vi "HFRR ADV v09.vi"() -> ()   [LabVIEW 2025] (continued)
18.549185433725157, 18.540397690756503, 18.52985239919411, 18.52985239919411, 18.5122769132568, 18.51403446185053, 18.515792010444265, 18.482398587163367, 18.494701427319487, 18.475368392788447, 18.464823101226052, 18.443732518101285, 18.459550455444862, 18.44900516388247, 18.427914580757704, 18.45076271247621, 18.436702323726358, 18.42439948357024, 18.433187226538898, 18.427914580757704, 18.408581546226657, 18.41385419200785, 18.389248511695616, 18.398036254664273, 18.38573341450815, 18.38221831732069, 18.38221831732069, 18.35058244263353, 18.368157928570838, 18.348824894039797, 18.34706734544607, 18.340037151071144, 18.331249408102487, 18.327734310915027, 18.31543147075891, 18.31543147075891, 18.301371082009055, 18.287310693259204, 18.297855984821588, 18.280280498884274, 18.275007853103087, 18.269735207321887, 18.25567481857205, 18.252159721384576, 18.232826686853535, 18.239856881228466, 18.215251200916224, 18.217008749509954, 18.209978555135034, 18.19064552060399, 18.195918166385184, 18.183615326229067, 18.169554937479216, 18.17307003466668, 18.153737000135635, 18.151979451541898, 18.137919062792054, 18.125616222635934, 18.12737377122967, 18.115070931073546, 18.115070931073546, 18.10276809091743, 18.099252993729966, 18.095737896542506, 18.09046525076131, 18.081677507792655, 18.067617119042804, 18.062344473261614, 18.055314278886687, 18.044768987324296, 18.03598124435564, 18.032466147168176, 18.023678404199522, 18.025435952793252, 18.021920855605796, 18.00961801544967, 17.99907272388729, 17.997315175293558, 17.99204252951236, 17.98501233513744, 17.97095194638759, 17.963921752012663, 17.958649106231476, 17.953376460450276, 17.946346266075352, 17.934043425919235, 17.93580097451296, 17.97095194638759, 17.953376460450276, 17.955134009044006, 17.94283116888789, 17.93931607170043, 17.927013231544308, 17.921740585763114, 17.891862259669683, 17.895377356857146, 17.89889245404461, 17.893619808263416, 17.881316968107296, 17.88307451670103, 17.879559419513566, 17.865499030763715, 17.833863156076553, 17.837378253264013, 17.80925747576432, 17.796954635608202, 17.796954635608202, 17.78465179545208, 17.77234895529596, 17.767076309514763, 17.777621601077154, 17.774106503889694, 17.742470629202533, 17.768833858108493, 17.719622497484025, 17.724895143265222, 17.724895143265222, 17.7178649488903, 17.728410240452682, 17.707319657327908, 17.70028946295298, 17.716107400296565, 17.703804560140444, 17.677441331234476, 17.65107810232851, 17.66865358826582, 17.5772610613918, 17.53859499232971, 17.52277705498613, 17.52453460357986, 17.515746860611202, 17.51047421483001, 17.50871666623628, 17.49992892326762, 17.491141180298964, 17.480595888736577, 17.477080791549124, 17.466535499986733, 17.464777951393007, 17.45423265983061, 17.44720246545569, 17.43314207670584, 17.43489962529957, 17.43138452811211, 17.419081687955984, 17.4085363963936, 17.403263750612407, 17.403263750612407, 17.390960910456286, 17.38744581326883, 17.382173167487633, 17.368112778737785, 17.368112778737785, 17.35405238998793, 17.347022195613008, 17.34174954983182, 17.339992001238087, 17.329446709675697, 17.325931612488237, 17.31714386951958, 17.308356126550922, 17.304841029363462, 17.303083480769722, 17.29429573780107, 17.278477800457495, 17.2732051546763, 17.26969005748884, 17.26265986311391, 17.257387217332717, 17.252114571551527, 17.245084377176603, 17.239811731395402, 17.23805418280167, 17.223993794051825, 17.223993794051825, 17.22047869686436, 17.213448502489445, 17.209933405301975, 17.20290321092705, 17.192357919364667, 17.188842822177204, 17.178297530614817, 17.17478243342735, 17.15720694749004, 17.146661655927648, 17.14490410733392, 17.136116364365265, 17.12908616999034, 17.122055975615414, 17.113268232646764, 17.178297530614817, 17.162479593271232, 17.115025781240494, 17.08338990655333, 17.081632357959595, 17.081632357959595, 17.067571969209745, 17.067571969209745, 17.06054177483482, 17.05702667764736, 17.051754031866164, 17.042966288897507, 17.035936094522594, 17.02363325436647, 17.01484551139781, 17.00957286561662, 16.995512476866768, 16.991997379679308, 16.990239831085574, 16.98496718530438, 16.979694539523184, 16.977936990929454, 16.96387660217961, 16.95508885921095, 16.951573762023486, 16.94278601905482, 16.933998276086164, 16.933998276086164, 16.92169543593005, 16.91642279014886, 16.9129076929614, 16.91642279014886, 16.904119949992744, 16.897089755617817, 16.895332207024087, 16.88654446405543, 16.87775672108677, 16.883029366867966, 16.867211429524385, 16.858423686555728, 16.85490858936826, 16.846120846399604, 16.832060457649764, 16.83030290905603, 16.823272714681107, 16.81624252030618, 16.810969874524982, 16.802182131556325, 16.8004245829626, 16.789879291400208, 16.789879291400208, 16.781091548431554, 16.768788708275437, 16.770546256869167, 16.767031159681704, 16.756485868119317, 16.754728319525583, 16.745940576556933, 16.738910382182006, 16.733637736400812, 16.724849993432162, 16.716062250463505, 16.702001861713647, 16.69672921593246, 16.698486764526187, 16.684426375776336, 16.682668827182606, 16.677396181401413, 16.666850889839022, 16.661578244057836, 16.659820695464106, 16.64927540390171, 16.640487660933058, 16.633457466558134, 16.628184820776944, 16.622912174995744, 16.622912174995744, 16.615881980620824, 16.60533668905843, 16.600064043277243, 16.59830649468351, 16.5807310087462, 16.577215911558728, 16.573700814371275]
  in  "ENTER THE NEW PASSWORD":string caption="Enter The New Password"
  in  "ENTER CURRENT PASSWORD":string caption="Enter Current Password"
  in  "Camera Port :":string(combo)="cam0"
  in  "Humidity :":refnum<visa-resource-name>="COM8"
  in  "LvdtOff":dbl=2.875 caption="LVDT Position Offset :" min=2.1 max=2.9 format="%.4f"
  out "Port 2 Error":errorcluster={"status"=TRUE, "code"=-1073807343, "source"="Property Node (arg 1) in VISA Configure Serial Port (Instr).vi->Winducom 2010--std ed hfrr-wo1768-V18.vi"}
  out "Port 1 Error":errorcluster={"status"=TRUE, "code"=-1073807343, "source"="Property Node (arg 1) in VISA Configure Serial Port (Instr).vi->Winducom 2010--std ed hfrr-wo1768-V18.vi"}
  in  "Stroke PID Gains":T8={"Proportional Gain (Kc)"=200.0, "Integral Time (Ti, min)"=0.02, "Derivative Time (Td, min)"=0.0}
  in  "CH-HUMIDITY DRY":u16=3 caption="Ch-Humidity Wet:" max=7 step=1
  in  "CH-HUMIDITY WET":u16=4 caption="Ch-Humidity Dry:" max=7 step=1
  in  "CH-HEATER":u16=2 caption="Ch-Heater:" max=7 step=1
  in  "CH-POWER -":u16=1 caption="Ch-Power -:" max=7 step=1
  in  "CH-POWER +":u16 caption="Ch-Power +:" max=7 step=1
  out "String 4":string
  in  "Prog Due":bool
  in  "Prog Uno":bool
  in  "Com Port 2":refnum<visa-resource-name>="COM7" caption="Port 2 :"
  in  "Com Port 1":refnum<visa-resource-name>="COM5" caption="Port 1 :"
  in  "Additional Parameter":T9(tab)
  out "CAMERA ROI MIN TEMP":bool
  in  "CAMERA ROI MAX TEMP":bool
  out "LIVE FEED MIN TEMP":bool
  in  "LIVE FEED MAX TEMP":bool
  in  "Temperature Off Command":bool
  in  "Temperature On Command":bool
  in  "Humidity Off Command":bool
  in  "Humidity On Command":bool
  out "Elapsed time":dbl caption="Elapsed Time" min=0.0 max=6000.0 step=0.01 format="%.2f"
  in  "Remaining Time":dbl min=0.0 max=180000.0 step=0.0001 format="%<%H:%M:%S>t"
  out "Auto Start Temp":bool
  out "Auto stop temp":bool
  in  "TestCompFlg":bool
  out "StartFlg":bool
  in  "Start Time":bool
  in  "sign in temp":bool
  in  "manual temp log":bool
  in  "Reach point temp":bool
  in  "Manual Humididty Reached":bool
  out "Humidity temp":dbl
  in  "Test ID":string
  in  "Reach point Humidity":bool
  in  "error in (no error) 2":errorcluster
  out "Instrument Status":bool=TRUE caption="Load COM Status"
  out "Heave Pulses/mm":dbl=1600.0
  out "Surge Pulses/mm":dbl=1600.0
  out "Sway Pulses/mm":dbl=320.0
  in  "Surge Pitch":dbl=3.0
  in  "Sway Pitch":dbl=2.0
  in  "Heave Pitch":dbl=4.0
  in  "Surge PPR":dbl=6400.0
  in  "Sway PPR":dbl=6400.0
  in  "Heave PPR":dbl=6400.0
  in  "Heater Trip Temp":bool
  out "String 41":string=":-@(Paltro : HIGH FREQUENCY RECIPROCATORY TEST RIG    DEFINITON FILE )      "
  out "Service Password enable":bool
  out "TEST FILE NAM,E SAVED":bool
  out "error out 6":errorcluster
  out "error out 7":errorcluster
  out "error out 8":errorcluster
  out "Camera List":string
  out "Image path  2":path caption="selected path"
  out "100x gain":dbl
  out "Pixel Value":dbl
  in  "Enum - Selector":T10
  out "Image path":path
  out "Error":errorcluster={"status"=TRUE, "code"=-1073807343, "source"="Property Node (arg 1) in VISA Configure Serial Port (Instr).vi->Winducom 2010--std ed hfrr-wo1768-V18.vi"}
  out "Bytes at Humidity Port":dbl
  in  "Com Port 4":refnum<visa-resource-name>="COM7" caption="COM Port Humidity :"
  out "Read Humidity":string
  in  "String 11":string
  in  "WriteHumidity":string[](array[string])
  out "LastCom":string
  in  "Write S":bool
  out "STALL :":string
  out "CURRENT :":string
  out "DEHUM :":string
  out "FAN_OUT :":string
  out "FAN_IN :":string
  out "PUMP :":string
  out "AMB_T :":string
  out "AMB_RH :":string
  out "T :":string
  out "RH :":string
  out "SET :":string
  out "STATE :":string
  out "RH Numeric:":dbl
  out "COM Status":bool=TRUE caption="Load COM Status"
  in  "Tab Control 6":enum32{"Data", "Sensor"}(tab)=enum."Sensor"
  out "Respose From Server":string
  out "standard output":string
  out "SinglePoint":string
  in  "JSON Check String":string="\"Stored\": true"
  in  "JSONH Check String":string="\"Stored\": true"
  out "standard output 2":string
  in  "Sensor Information":string[][](array[string])=[["Sensor Name", "Sensor Model Number", "Sensor Run time Hours", "Sensor State"], ["Normal Load Sensor", "MPF-AC20-X3U791", "", ""], ["Frictional Force Sensor", "MPF-AC20-X3U792", "", ""], ["Temperature Sensor", "MPF-AC20-X3U793", "", ""], ["Speed Sensor", "MPF-AC20-X3U794", "", ""], ["LVDT Sensor", "MPF-AC20-X3U795", "", ""], ["Vibration Sensor ", "MPF-AC20-X3U796", "", ""]]
  out "Respose From Server 2":string
  in  "Total No. of Tests":dbl
  in  "Upld AR":bool
  in  "Sensor File Name":string="JSON_Health.JSON"
  in  "Run test 3":bool
  in  "Sen.Upload Rate (s)":dbl=5.0 min=0.5 max=5.0 step=0.5 format="%.1g"
  in  "Upld AR 2":bool
  in  "Path":path=path "C:/LAB-IQ-NXT"
  in  "Data File Name":string="JSON_Single_Point.JSON"
  in  "Model No":string="MD987654325"
  in  "Serial No":string="HFRR2391"
  in  "Secret Key":string="22gKHnAGFaJhuNtaR9srYhcD6RQR8M7Zp2xk4ssPTuwGqWUBv7WxW7cXAFkFFbns"
  in  "Upload Rate (s)":dbl=1.0 min=0.5 max=5.0 step=0.5 format="%.1g"
  in  "ADC Res":u16(ring) items=["16 bit", "24 bit"]
  out "Test Standard":string
  out "error out 5":errorcluster
  out "after substring":string
  out "before substring 2":string
  in  "Temperature after test 3":dbl caption="Temp After Test" format="%#_5g"
  in  "Humidity after test 3":dbl caption="Humidity After Test" format="%#_5g"
  in  "Tab Control 4":T11(tab)=enum."Temperature Tuning"
  in  "ECR_Gain":dbl=24000.0
  out "Ch3 2":dbl[](graph)
  out "Air temp":dbl[](graph)
  out "ECR":dbl[](graph)
  out "Rtemp":dbl[](graph)
  in  "Do 0":bool
  out "DI 0":bool=TRUE
  out "DI 1":bool=TRUE
  out "DI 2":bool=TRUE
  out "DI 3":bool=TRUE
  out "DI 4":bool=TRUE
  out "DI 5":bool=TRUE
  out "DI 6":bool=TRUE
  out "DI 7":bool=TRUE
  in  "Do 7":bool
  in  "Do 6":bool
  in  "Do 5":bool
  in  "Do 4":bool
  in  "Do 3":bool
  in  "Do 2":bool
  in  "Do 1":bool
  in  "output range":cluster{"output high":dbl, "output low":dbl}={"output high"=110.0, "output low"=0.0}
  in  "Offset Air Temp":dbl
  in  "Temp PID gains":T12={"proportional gain (Kc)"=10.0, "integral time (Ti, min)"=1.66, "derivative time (Td, min)"=0.0}
  out "gTEMP 3":cluster{dbl, "output":dbl, "Set Temp":dbl}(graph)={6.858462627117447, "output"=42.16277107130474, "Set Temp"=53.14153737288255}
  out "Pk-Pk":dbl=0.5
  in  "Offset":dbl=0.5
  in  "Gain":dbl=1.4
  out "gLVDTraw":dbl[](graph)
  out "Disp":dbl=-1.7485910993892546e-16 caption="Stroke" format="%.2f"
  out "Freq":dbl=50.0 caption="Frequency" min=10.0 max=250.0 step=0.1 format="%.2f"
  out "PID Out":u8(slide) scale=0.0..4095.0
  out "Freq":dbl min=0.0 max=12.0 step=0.01 format="%.3f"
  out "Array":string[](array[string])
  out "UnoRead":string
  out "Sps 2":dbl=890.0 format="%_0f"
  out "Disp (mm)":dbl=1.0 min=0.0 max=12.0 step=0.01 format="%.3f"
  in  "PID Rst":bool=TRUE
  in  "DC correction":bool=TRUE
  out "Mean(RAW) Stroke":dbl(graph)
  out "Waveform Graph 2":waveform(dbl)[](graph)
  out "Stroke PID OUT":dbl(slide)=-13.483146067415703 scale=-600.0..600.0
  out "Slide 8":cluster{dbl, dbl, dbl}(slide)={-13.483146067415703, -400.0, -400.0} scale=-0.8..0.8
  in  "Tab Control 8":enum32{"setup", "calibrate"}(tab)
  in  "Boolean 10":bool
  in  "Measure":bool
  in  "Measure 2":bool
  in  "Boolean 11":bool
  in  "Zero 4":bool
  out "Intercept":dbl
  out "Slope":dbl
  in  "Captured Values 2":dbl[][](array[numeric])
  in  "Zero 3":bool
  out "software msrnt":dbl=50.0 caption="Software measurment" min=0.0 max=250.0 step=0.001 format="%.4f"
  out "Measure_LDS":dbl=50.0 caption="Position (high precision laser)" min=0.0 max=250.0 step=0.001 format="%.4f"
  in  "Boolean 9":bool
  in  "Boolean 8":bool
  in  "Boolean 7":bool
  out "?":cluster{"Y":dbl[], "Y":dbl[]}[](graph)
  in  "Laser Disp Sensor":refnum<visa-resource-name>="COM14" caption="COM Port"
  in  "COMMAND":string="OUTPUT RS422"
  in  "COMMAND 2":string="OUTPUT NONE\n"
  in  "ACQUIRE 2":bool
  out "Friction Force (N)":ext=1.0 format="%_4f"
  out "G_val":dbl
  out "Current (A)":ext=1.0 format="%_4f"
  in  "Window":ext=1.0
  out "Constant (G)":dbl(graph)
  out "Waveform Graph 4":dbl[][](graph)
  in  "Humidity BaudRate":dbl=9600.0
  in  "Re-Initialise":bool
  out "Humidity 2":u32(graph)
  out "Port 2":u32(graph)
  out "Port 1":u32(graph)
  out "autostrtflg":bool
  out "airtempflg":bool
  out "z_measure":dbl
  in  "ACQUIRE 3":bool
  out "pk-pk":cluster{dbl, "t":dbl}(graph)
  out "Read String":string
  out "Waveform Graph 5":dbl[](graph)
  out "Waveform Chart 3":dbl[](graph)
  out "set temp old":dbl
  out "Error Code":errorcluster
  in  "Rd":bool
  out "String 10":string
  in  "Length 2":i16=16 caption="Set" min=1 max=60 step=1
  out "path 2":path
  out "image data":T13
  out "new picture":picture
  out "error out 2":errorcluster
  out "String Indicator 4":string
  out "String Indicator 3":string
  in  "OPEN 5":bool
  out "string1 5":string
  out "String 49":string="Tested by"
  out "String 48":string="Sample ID "
  out "String 47":string="Tested date"
  out "String 46":string="S.NO"
  out "test by 2":string
  in  "ISO : WS1.4":enum32{"Page 1", "Page 2"}(tab)
  in  "Save Results":bool
  out "String 23":string="ISO : WS1.4"
  out "Rh After":dbl min=0.0 max=100.0 step=1.0 format="%.1f"
  out "Rh Before":dbl min=0.0 max=100.0 step=1.0 format="%.1f"
  in  "Humidity before test":dbl min=0.0 max=100.0 step=1.0
  out "AVP":dbl=0.0032746494993313616 format="%.3f"
  in  "MWSD":dbl
  out "WS1.4":dbl format="%1.2f"
  in  "HCF":dbl min=0.0 max=10000.0 step=0.01 format="%.2f"
  in  "Temperature before test":dbl=1.0 caption="Temp before test" min=1.0 max=100.0 step=0.1 format="%.1f"
  in  "Humidity after test":dbl=1.0 min=1.0 max=100.0 step=1.0
  in  "Temperature after test":dbl=1.0 caption="Temp after test" min=1.0 max=100.0 step=0.1 format="%.1f"
  out "WS1.4 2":dbl caption="WS1.4" format="%#_5g"
  out "HCF 2":dbl caption="HCF" format="%#_5g"
  out "AVP 2":dbl caption="AVP" format="%#_5g"
  out "MWSD 2":dbl caption="MWSD" format="%#_5g"
  out "Temperature after test 2":dbl caption="Temp after test" format="%#_5g"
  out "Humidity after test 2":dbl caption="Humidity after test" format="%#_5g"
  out "Temperature before test 2":dbl caption="Temp before test" format="%#_5g"
  out "Humidity before test 2":dbl caption="Humidity before test" format="%#_5g"
  out "Voltage LVDT Acq":dbl[](graph)
  out "Stroke_send_Val":string
  out "AirT":dbl(graph)
  out "temp_@Rh sensor":string
  out "refresh flag":bool
  out "Air temp":string
  in  "hide controller":enum32{"Hidden", "controllers"}(tab)=enum."controllers"
  in  "UUID":string caption="UUID    :"
  in  "FLAG 4":dbl min=0.0 max=999999999.0 step=0.25 format="%.2f"
  out "START 3":dbl format="%.1f"
  in  "FLAG 2":dbl min=0.0 max=999999999.0 step=0.25 format="%.2f"
  out "JSON string":string
  out "Sensor Health JSON string":string
  out "run replace":bool
  out "cof":dbl caption="Frictional Torque" format="%.2f"
  out "time":dbl caption="Time \nRemaining"
  out "SEN.RUN HRS":dbl
  out "Json St Flg":bool
  out "Json End Flg":bool
  out "temp_st":string
  out "sp_st":string
  out "FF STATE":i32
  out "nlstate":string
  out "ffstate":string
  out "nl_st":string
  out "ff_st":string
  in  "in":string[](array[string])=["", "", "", "", "", "", ""]
  out "out":string[](array[string])=["Sensor State", "", "", "", "", "", ""]
  out "SinglePoint  2":string
  out "Sensor name":string[](array[string])
  out "model num":string[](array[string])
  out "run time":string[](array[string])
  out "state":string[](array[string])
  out "state1":string[](array[string])
  out "T cycle":dbl caption="TOTAL\nTIME"
  in  "Length":i16=16 caption="Set" min=1 max=60 step=1
  out "acq 2":bool
  out "Stroke Ln 2":string
  out "St Str":string
  out "run":string[](array[string])
  out "ecr 2":dbl caption="Pin temp"
  out "run hrs":string
  in  "tfalg":dbl
  out "Temp":dbl caption="Pin temp"
  in  "yflag":dbl
  in  "zflag":dbl
  out "zflag 2":dbl
  out "Stroke Ln":dbl caption="Normal Load"
  out "SENSOR TIME":dbl
  out "TEMP STATE":i32
  out "NL STATE":i32
  in  "FLAG":dbl min=0.0 max=999999999.0 step=0.25 format="%.2f"
  out "START 2":dbl format="%.1f"
  out "SENSOR TIME  2":dbl
  out "Rt 3":bool
  out "Rt":bool
  out "Rt 2":bool=TRUE
  in  "Reset 4":bool caption="Reset"
  in  "tmpchk":bool
  out "Temp ini":dbl min=0.0 max=150.0 step=1.0
  in  "wait":u32=1000
  out "humid":string
  out "Ser Led":bool
  in  "Send":bool
  out "Humidity Str Rec":string
  in  "Humidity Str Send":string="stop"
  out "String 9":string
  in  "Reset 3":bool caption="Reset"
  in  "check time s":dbl=10.0
  in  "Threshold value":dbl=1000.0
  out "file count":i32
  out "Waveform Graph":dbl[][](graph)
  in  "Hold 4":bool
  in  "save dpt":bool
  in  "FILE 2":string="Spike Cpture" caption="File name"
  out "Humid Last buf":dbl[](graph)
  out "visa due":string(combo)="COM63" caption="Visa Module 2 ( Due )"
  in  "Tab Control":T14(tab)
  in  "Info Square":bool
  out "String 43":string="mm"
  in  "Home 8":bool
  in  "Home 9":bool
  out "String 18":string="min"
  out "String 22":string="min"
  out "String 17":string="Timer"
  in  "Samplingtime 2":dbl=0.5 caption="Save Dwell" min=0.1 max=600.0 step=0.1 format="%.1g"
  out "String 21":string="Sec"
  in  "RST FF":bool
  in  "RSTCOF 3":bool
  in  "RST TEMP":bool
  in  "RSTCOF":bool
  in  "Home":bool caption="Password"
  in  "Configure":bool caption="Password"
  in  "Analysis 2":bool caption="Password"
  in  "service 3":bool caption="Password"
  in  "EXIT 2":bool
  in  "GRAY SCALE INTERCHANGE":enum32{"GRAY IMAGE", "RGB IMAGE"}(radio)=enum."RGB IMAGE"
  in  "Lubrication System COM Port :":refnum<visa-resource-name>="COM9" caption="Ambient Temperature COM Port:"
  in  "Com Port 3":refnum<visa-resource-name>="COM4" caption="Port 3"
  in  "STOP 2":bool
  out "Upload \nConfirmed 2":bool caption="Health"
  out "Upload \nConfirmed":bool caption="Data"
  out "AR Led":bool caption="AR"
  in  "autostart":bool caption="RUN"
  in  "SetTemp 2":dbl=23.0 caption="Set" min=1.0 max=26.0 step=1.0
  out "autostart 2":string
  out "String 14":string
  out "TK4 status":bool=TRUE caption="Air Status"
  in  "Heater":bool
  out "Amb temp":dbl caption="Air Temperature" min=0.0 max=150.0 step=1.0 format="%.1f"
  out "SetTemp":dbl=23.0 caption="Set" min=20.0 max=26.0 step=1.0
  in  "Engage":bool
  out "Countdown 2":dbl caption="Present ( Sec )" min=1.0 max=6000.0 step=1.0
  in  "Countdown":dbl=1.0 caption="Count down ( Sec )" min=1.0 max=6000.0 step=1.0
  in  "PWR":bool
  in  "st enable":bool
  out "COF - filtered":dbl min=0.0 max=200.0 step=0.1 format="%.2f"
  in  "% Humidity":dbl=35.0 min=1.0 max=100.0 step=1.0
  out "Peak - Peak 2":dbl
  out "COF":dbl=100.0 min=0.0 max=200.0 step=0.1 format="%.1f"
  out "act save time":dbl=3561152582.7339997 format="%.2f"
  out "acq timer":dbl=3614575087.823 format="%.2f"
  out "Cycles elapsed":i32=5
  in  "Save":bool
  out "cyclecount":i32
  out "speedop":dbl min=0.0 max=999999999.0 step=0.25 format="%.2f"
  out "cmp":i32
  in  "OPEN 6":bool
  out "freq1":dbl format="%_4f"
  out "freq2":dbl format="%_4f"
  out "freq3":dbl format="%_4f"
  out "sample1":dbl format="%_4f"
  out "sample2":dbl format="%_4f"
  out "sample3":dbl format="%_4f"
  out "String 6":string="  "
  in  "String 7":string="  "
  out "String 12":string="  "
  out "String 8":string="  "
  out "Numeric 13":i32
  out "Numeric 12":i32
  out "Numeric 11":i32
  out "Numeric 8":i32
  in  "Ref B Scar Value :":string caption="Reference Fluid Information"
  in  "Ref B Test Date :":string caption="Reference Fluid Information"
  in  "Ref A Scar Value :":string caption="Reference Fluid Information"
  in  "Image Path":path
  in  "Wear Scar Y":dbl caption="Wear Scar Minor Axis ( Microns )" format="%#_5g"
  in  "Wear Scar X":dbl caption="Wear Scar Major Axis ( Microns )" format="%#_5g"
  in  "Print 2":bool caption="Печать"
  in  "Ref A Test Date :":string caption="Reference Fluid Information"
  out "XY Graph 17":cluster{dbl[], dbl[]}[](graph)
  in  "Print 3":bool caption="Печать"
  in  "Select File Type":enum16{"xlx", "csv", "txt"}(ring)
  out "s.NO":string caption="S.NO"
  in  "Export":bool
  out "Test Date":string caption="Tested date"
  out "Tested by":string
  out "Sample ID":string
  in  "OK Button 16":bool
  out "String Indicator":string
  out "String Indicator 2":string
  in  "OK Button 17":bool
  out "Selected Printer":string="Microsoft XPS Document Writer"
  in  "Select Printer 3":i32 caption="Select Printer"
  out "System Configured Printers 2":string[](array[string])=["Microsoft XPS Document Writer", "Fax", "CutePDF Writer", "\\\\192.168.1.28\\RICOH Aficio MP 2352 PCL 6"] caption="System Configured Printers"
  out "TITTLE":string caption="Tittle"
  in  "Sample ID  5":string caption="Fuel S/N:"
  in  "Sample ID  4":string caption="Fuel Name:"
  in  "Sample ID  3":string caption="Fuel Type:"
  in  "Print":bool caption="Печать"
  in  "SPEED OUT:":dbl=1.0 caption="Speed Out:" min=0.0001 max=5.0 step=0.0001 format="%.4f"
  in  "Temperature before test 3":dbl caption="Temp Before Test" format="%#_5g"
  in  "Humidity before test 3":dbl caption="Humidity Before Test" format="%#_5g"
  out "Temperature after test 5":dbl caption="Temp Before Test" format="%#_5g"
  out "Temperature after test 4":dbl caption="Temp After Test" format="%#_5g"
  out "Humidity after test 4":dbl caption="Humidity After Test ( % Rh )" format="%#_5g"
  out "Humidity before test 4":dbl caption="Humidity Before Test ( % Rh )" format="%#_5g"
  in  "Tab Control 9":enum32{"Page 1", "Page 2"}(tab)
  out "Ref B Scar Value :":string caption="Reference Fluid Information"
  out "Ref B Test Date :":string caption="Reference Fluid Information"
  out "Ref A Scar Value :":string caption="Reference Fluid Information"
  out "Ref A Test Date :":string caption="Reference Fluid Information"
  out "XY Graph 16":cluster{dbl[], dbl[]}[](graph)
  out "TITTLE 4":string caption="Reference Fluid Information"
  out "Sample ID  7":string caption="Fuel Name :"
  out "Sample ID  6":string caption="Fuel Type :"
  out "Mean Wear ( microns) :":dbl format="%#.6f"
  out "Wear Scar Y ( microns ) :":dbl format="%#.6f"
  out "Length ( microns ) 2":dbl caption="Wear Scar X ( microns ) :" format="%#.6f"
  out "s.NO 2":string caption="Instrument  S.NO :"
  out "Test Date 2":string caption="Tested date :"
  out "Tested by 2":string caption="Tested by :"
  out "Sample ID  2":string caption="Sample ID :"
  out "TITTLE 2":string caption="File Name :"
  in  "EDIT 3":bool
  out "FF buffer":dbl[](graph)
  out "%  o/p":dbl
  out "sample4":dbl format="%_4f"
  out "freq 4":dbl format="%_4f"
  out "conststatus":dbl=10.0 min=0.0 max=200.0 step=1.0
  out "CP4":dbl=nan min=0.0 max=200.0 step=0.1 format="%.3f"
  out "CP3":dbl=nan min=0.0 max=200.0 step=0.1 format="%.3f"
  out "Boolean  4":bool=TRUE caption="Power Status"
  in  "Boolean BC T & BG 2":cluster{u32, u32}[](array[cluster])=[{3158064, 16250871}, {11918296, 8965631}]
  in  "GBG   2":u32(colorbox)=16250871 caption="Graph Background"
  in  "GFG  2":u32(colorbox)=8964095 caption="Graph Foreground"
  in  "GBG":u32(colorbox)=16250871 caption="Graph Background"
  in  "GFG":u32(colorbox)=8964095 caption="Graph Foreground"
  in  "Boolean BC T & BG":cluster{u32, u32}[](array[cluster])=[{3158064, 16250871}, {11918296, 8965631}]
  in  "SC  Text":u32(colorbox) caption="String Control Text"
  in  "SC BG 3":u32(colorbox)=16777215 caption="String Control BG"
  in  "NI BG 2":u32(colorbox)=13553358 caption="Numeric Indicator BG"
  in  "NI Text  2":u32(colorbox)=7105644 caption="Numeric Indicator Text"
  in  "NC Text":u32(colorbox)=3381759 caption="Numeric Control Text"
  in  "NC BG":u32(colorbox)=16777215 caption="Numeric Control BG"
  out "ABS DP":dbl[](graph)
  in  "Com flag":u32
  out "Gain path":string="C:\\Winducom 2010\\STD ED HFRR\\wo1768"
  out "String 45":string="S.NO"
  out "String 44":string
  out "error out 4":errorcluster
  out "concatenated string 2":string
  out "String 42":string
  out "error out 3":errorcluster
  out "STR":string
  out "gain":string
  out "export":string
  out "before substring":string
  out "output":string
  out "test by":string
  out "export 2":string
  out "export":string
  out "REMARKS 2":string="@WINDUCOM : RECIPROCATORY TEST RIG    DEFINITON FILE       \r  Sample ID :- , Load :-  2.00 N , Remarks :- , Date :- 05/11/2016, 06:04\r"
  out "data":string
  out "Boolean 3":bool
  out "concatenated string":string
  out "path":path
  out "String 40":string
  out "Boolean 2":bool=TRUE
  in  "Set Rh 2":dbl=50.0 caption="HUMIDITY" min=35.0 max=85.0 step=1.0
  out "String 39":string="WS1.4="
  out "String 38":string="HCF="
  out "String 37":string="MWSD="
  out "String 36":string="AVP ="
  out "String 35":string="Temp after test="
  out "String 34":string="Temp before test="
  out "String 33":string="Tested by"
  out "String 32":string="Sample ID "
  out "String 31":string="Tested date"
  out "String 30":string="Sample Design"
  out "path string":string
  out "String 29":string
  out "St. Line eqn : 2":string
  out "Numeric 10":i32
  out "Numeric 16":i32
  out "S 106":string="Off"
  out "S 105":string="On"
  out "S 104":string="Heater Off"
  out "S 103":string="Heater On"
  out "S 102":string="Ch-Humidity Dry:"
  out "S 101":string="Ch-Humidity Wet:"
  out "S 100":string="Ch-Heater:"
  out "S 99":string="Ch-Power -:"
  out "S 98":string="Ch-Power +:"
  out "S 97":string="Port 2"
  out "S 96":string="Port 1"
  out "S 95":string="Stroke Gain :"
  out "S 94":string="Displacement :"
  out "S 93":string="Stop"
  out "S 92":string="Run"
  in  "LAnguage":enum32{"Page 1", "Page 2"}(tab)
  out "S 91":string="Threshold"
  out "S 90":string="File path"
  out "S 89":string="Newtons ( N )"
  out "S 88":string="Change Calibrate Password"
  out "S 87":string="Enter The New Password"
  out "S 86":string="Enter Current Password"
  out "S 85":string="Password"
  out "S 84":string="Save Gain Constants"
  out "S 83":string="Air Temperature ( deg C )"
  out "S 82":string="TIME ( mins )"
  out "S 81":string="Relative Humidity ( Rh )"
  out "S 80":string="Sample TEMPERATURE ( Deg C)"
  out "S 79":string="Stroke"
  out "S 78":string="Air Temperature"
  out "S 77":string="mm"
  out "S 76":string="Stroke"
  out "S 75":string="WINDUCOM 2010 \\XXXX\\VX.XX\\MONTH YEAR"
  out "S 74":string="Frictional Force ( N )"
  out "S 73":string="Calibrate Parameter"
  out "S 72":string="Save Gain Constant"
  out "S 71":string="Edit Gain Constant"
  out "S 70":string="Humidity :"
  out "S 69":string="Air Temperature :"
  out "S 68":string="Speed Out:"
  out "S 67":string="Temperature :"
  out "S 66":string="Frictional Force :"
  out "S 65":string="ABOUT"
  out "S 64":string="Frictional  Force ( N )"
  out "S 63":string="Temperature ( Deg C)"
  out "S 62":string="Time ( mins )"
  out "S 60":string="Reset Graph"
  out "S 59":string="COF4"
  out "S 58":string="COF3"
  out "S 57":string="COF2"
  out "S 56":string="COF1"
  out "S 55":string="Frictional Force ( N )"
  out "S 54":string="Temperature"
  out "S 53":string="Coefficient Of Friction"
  out "S 52":string="Refresh"
  out "S 51":string="File 4"
  out "S 50":string="File 3"
  out "S 49":string="File 2"
  out "S 48":string="File 1"
  out "S 47":string="COMPARE FILES"
  out "S 46":string="SAVE RESULT"
  out "S 45":string="WS1.4"
  out "S 44":string="HCF"
  out "S 43":string="MWSD"
  out "S 42":string="AVP "
  out "S 41":string
  out "S 40":string
  out "S 39":string="Humidity after test="
  out "S 38":string="Humidity before test="
  out "S 37":string
  out "S 36":string="Rh Before"
  out "S 35":string="ISO : WS1.4"
  out "S 34":string="FRICTIONAL FORCE ( N )"
  out "S 33":string="Reset Graph"
  out "S 32":string="Data points"
  out "S 31":string="COEFFICIENT OF FRICTION"
  out "S 30":string="RUN"
  out "S 29":string="Test Status"
  out "S 28":string="Power"
  out "S 27":string="Engage"
  out "S 26":string="Present ( Sec )"
  out "S 25":string="Count down ( sec )"
  out "S 24":string="Sec"
  out "S 23":string="Save Dwell"
  out "S 22":string="Elapsed Time"
  out "S 21":string="min"
  out "S 20":string="Test duration"
  out "S 19":string="TIMER"
  out "S 18":string="OFF"
  out "S 17":string="Rh"
  out "S 16":string="HUMIDITY"
  out "S 15":string="Heater On"
  out "S 14":string="TEMPERATURE ( Deg C)"
  out "S 13":string="N"
  out "S 12":string="NORMAL LOAD"
  out "S 11":string="Hz"
  out "S 10":string="FREQUENCY"
  out "S 9":string="STOP"
  out "S 8":string="STAND BY"
  out "S 7":string="Remarks :"
  out "S 6":string="Sample ID :"
  out "S 5":string="File Name :"
  out "S 4":string="Acquire"
  out "S 3":string="EXIT"
  out "S 2":string="Winducom 2010"
  out "S":string="ENGLISH TITLES"
  out "Error Due":errorcluster={"status"=TRUE, "code"=-1073807343, "source"="Property Node (arg 1) in VISA Configure Serial Port (Instr).vi->Winducom 2010--std ed hfrr-wo1768-V18.vi"}
  out "Error Uno":errorcluster={"status"=TRUE, "code"=-1073807343, "source"="Property Node (arg 1) in VISA Configure Serial Port (Instr).vi->Winducom 2010--std ed hfrr-wo1768-V18.vi"}
  out "as":string
  out "bs":string="Rh After"
  out "as":string=" after test"
  out "bs":string="Temp"
  out "as":string=" before test"
  out "bs":string="Temp"
  out "as":string=" after test"
  out "bs":string
  out "bs":string="Humidity"
  out "as":string=" before test"
  out "bs":string="Humidity"
  out "S 61":string="Frictional Force ( N )"
  in  "Lan flag":dbl=22.0
  in  "Table":string[][](table)=[["ENGLISH TITLES", "RUSSIAN"], ["Winducom 2010", "Winducom  2010"], ["Exit", "Выход"], ["Acquire", "ИСПЫТАНИЕ     "], ["File Name :", "Имя файла :"], ["Sample ID :", "Имя образца :"], ["Remarks :", "Примечания :"], ["Standby", "ОЖИДАНИЕ"], ["Stop", "СТОП"], ["Frequency", "ЧАСТОТА"], ["Hz", "Гц"], ["Normal Load", "НАГРУЗКА"], ["N", "Н"], ["Temperature ( Deg C)", "ТЕМПЕРАТУРА (Град С)"], ["Heater On", "НАГРЕВ ВКЛ"], ["Humidity", "ВЛАЖНОСТЬ"], ["Rh", "%"], ["OFF", "ВЫКЛ"], ["Timer", "ВРЕМЯ"], ["Test duration", "ВРЕМЯ ТЕСТА"], ["min", "мин"], ["Elapsed Time", "依商判"], ["Save Dwell", "ИНТЕРВАЛ"], ["Sec", "Сек"], ["Count down ( Sec )", "До запуска (сек)"], ["Present ( Sec )", "Таймер (сек)"], ["Run", "Применить"], ["Power", "ПИТАНИЕ"], ["Test Status", "СТАТУС"], ["Manual Over Ride", "ПУСК"], ["Coefficient Of Friction", "КОЭФФИЦИЕНТ ТРЕНИЯ"], ["Data points", "Точки"], ["Reset Graph", "Сбросить график"], ["Frictional Force ( N )", "СИЛА ТРЕНИЯ (Н)"], ["ISO : WS1.4", "ISO : WS1.4"], ["Rh Before", "Влажность до"], ["Rh After", "Влажность, после"], ["Humidity, before test", "Влажность, до теста"], ["Humidity, after test", "Влажность, после теста"], ["Temp, before test", "Температура, до теста"], ["Temp, after test", "Температура, после теста"], ["AVP ", "СДП"], ["MWSD", "MWSD"], ["HCF", "ФКВ"], ["WS1.4", "WS1.4"], ["Save Result", "Сохранить результат"], ["COMPARE FILES", ""], ["File 1", "ФАЙЛ 1"], ["File 2", "ФАЙЛ 2"], ["File 3", "ФАЙЛ 3"], ["File 4", "ФАЙЛ 4"], ["Refresh", "ОБНОВИТЬ"], ["Coefficient Of Friction", "КОЭФФИЦИЕНТ ТРЕНИЯ"], ["Temperature", "ТЕМПЕРАТУРА"], ["Frictional Force ( N )", "СИЛА ТРЕНИЯ (Н)"], ["COF1", "КОФ1"], ["COF2", "КОФ2"], ["COF3", "КОФ3"], ["COF4", "КОФ4"], ["Reset Graph", "Сбросить график"], ["Time ( mins )", "Время (мин)"], ["Temperature ( Deg C)", "ТЕМПЕРАТУРА (Град С)"], ["Frictional  Force ( N )", "СИЛА ТРЕНИЯ (Н)"], ["ABOUT", ""], ["Frictional Force :", "КОЭФ.ТРЕНИЯ:"], ["Temperature :", "ТЕМПЕРАТУРА"], ["Speed Out:", "СКОРОСТЬ"], ["Air Temperature :", "ТЕМПЕРАТУРА ВОЗДУХА"], ["Humidity :", "ВЛАЖНОСТЬ"], ["Edit Gain Constant", "КОРРЕКТИРОВКА КОНСТАНТ"], ["Save Gain Constant", "СОХРАНИТЬ КОНСТАНТЫ"], ["Calibrate Parameter", "ПАРАМЕТРЫ КАЛИБРОВКИ"], ["Frictional Force ( N )", "СИЛА ТРЕНИЯ (Н)"], ["WINDUCOM 2010 \\XXXX\\VX.XX\\MONTH YEAR", "WINDUCOM 2010 \\XXXX\\VX.XX\\MONTH YEAR"], ["Stroke", "ДЛИННА ХОДА"], ["mm", "мм"], ["Air Temperature", "ВОЗДУХА ТЕМП"], ["Stroke", "ДЛИННА ХОДА "], ["Time ( mins )", "ВРЕМЯ ( мин )"], ["Sample Temperature( Deg C)", "Образец ТЕМПЕРАТУРА (Град С)"], ["Relative Humidity ( Rh )", "Относительный Влажность ( % )"], ["Air Temperature ( deg C )", "ТЕМПЕРАТУРА ВОЗДУХА (Град С)"], ["Save Gain Constants", "СОХРАНИТЬ КОНСТАНТЫ"], ["Password", "ПАРОЛЬ ДОСТУПА"], ["Enter Current Password", "ВВЕДИТЕ ТЕКУЩИЙ ПАРОЛЬ"], ["Enter The New Password", "ВВЕДИТЕ НОВЫЙ ПАРОЛЬ"], ["Change Calibrate Password", "Сбросить пароль калибровки"], ["Newtons ( N )", "Ньютон ( Н )"], ["File path", "Путь к файлу"], ["Threshold", "порог"], ["Run", "ПУСК"], ["Stop", "СТОП"], ["Displacement :", "смещение:"], ["Stroke Gain :", "ДЛИННА ХОДА:"], ["Port 1", "порт 1"], ["Port 2", "порт 2"], ["Ch-Power +:", "CH-ПИТАНИЕ +:"], ["Ch-Power -:", "CH-ПИТАНИЕ -:"], ["Ch-Heater:", "НАГРЕВ:"], ["Ch-Humidity Wet:", "CH-Увлажнение:"], ["Ch-Humidity Dry:", "CH-Осушение:"], ["Heater On", "НАГРЕВ ВКЛ"], ["Heater Off", "НАГРЕВ ВЫКЛ"], ["On", "ВКЛ"], ["Off", "ВЫКЛ"], ["TEXT REPORT", "ПРОТОКОЛ ИСПЫТАНИЯ"], ["Open Data File", "ОТКРЫТЬ ФАЙЛ ДАННЫХ"], ["Refresh", "ОБНОВЛЕНО"], ["Tittle", "заглавие"], ["Sample Design", "Образец"], ["Tested date", "Дата"], ["Sample ID ", "Имя образца"], ["Tested by", "Испытано"], ["System Configured Printers ", "Сконфигурированные принтеры"], ["Selected Printer", "Выбранный принтер"], ["Select Printer 3", "Выбрать  Печать"], ["Print", "Печать"], [":-@(WINDUCOM : RECIPROCATORY TEST RIG    DEFINITON FILE )      ", "(Анализатор HFRR с возвратно-поступательным механизмом для определения смазывающей способности дизельных топлив )"], ["Tested by:", "Оператор:"], ["          TIME;      COF;       STROKE  (mm);     AIR TEMP ( Deg C);  TEMP ( Deg C);  HUMIDITY ( Rh );", "КОЭФФИЦИЕНТ ТРЕНИЯ;   Инсульт; ТЕМПЕРАТУРА ВОЗДУХА; ВЛАЖНОСТЬ;"], ["Export", "Экспорт"], ["Temperature Intercept :", "ТЕМП перехват:"], ["Air Temperature Intercept:", "ТЕМП  ВОЗДУХА перехват:"], ["Select File Type ", "Выберете формат файла"], ["S.NO", "S.NO"], ["Trip", ""]]
  out "Fric Val":dbl[](array[numeric])
  out "FF cal val":dbl[](array[numeric])=[-0.013084344151737926, -0.01288606647100253, -0.011498122705853597, -0.012092955748060075, -0.011101567344382515, -0.011696400386589284, -0.010705011982911433, -0.010110178940704664, -0.011498122705853597, -0.01090328966364712, -0.009911901259969269, -0.009911901259969269, -0.009515345898498478, -0.008523957494820628, -0.008127402133349837, -0.008127402133349837, -0.009118790537027396, -0.008325679814085232, -0.008325679814085232, -0.008523957494820628, -0.008325679814085232, -0.008127402133349837, -0.008523957494820628, -0.00792912445261415, -0.008325679814085232, -0.008325679814085232, -0.007730846771878755, 0.0015882042226915277, -0.0027739047534900835, -0.0059463476452584485, -0.007136013729671986, -0.006739458368200904, -0.008325679814085232, -0.008523957494820628, -0.007334291410407381, -0.007730846771878755, -0.007334291410407381, -0.007136013729671986, -0.00792912445261415, -0.007334291410407381, -0.006937736048936299, -0.006342903006729822, -0.006342903006729822, -0.006342903006729822, -0.006144625325994427, -0.006144625325994427, -0.0055497922837873664, -0.004954959241580889, -0.005351514603051971, -0.004954959241580889, -0.004954959241580889, -0.004161848518639016, -0.003170460114961457, -0.0023773493920190014, -0.0023773493920190014, -0.0019807940305479194, -0.0019807940305479194, -0.0011876833076060467, -0.0009894056268700685, -0.0009894056268700685, -0.0009894056268700685, -0.0007911279461346732, -0.00019629490392819582, 0.00020026045754288624, 0.0007950934997493636, 0.001389926541955841, 0.0021830372648982965, 0.0033727033493112513, 0.004165814072253707, 0.0037692587107826248, 0.0037692587107826248, 0.004165814072253707, 0.0049589247951955795, 0.005752035518137744, 0.006346868560344221, 0.007338256964022072, 0.007734812325493154, 0.008726200729171005, 0.010510699855790728, 0.00991586681358396, 0.011105532897997497, 0.011502088259468288, 0.012096921301675348, 0.012493476663146139, 0.01289003202461722, 0.01289003202461722, 0.014277975789765862, 0.015269364193443713, 0.016260752597121272, 0.01745041868153452, 0.018243529404476683, 0.019036640127418555, 0.018640084765947473, 0.01982975085036101, 0.020028028531096406, 0.021415972296245048, 0.021415972296245048, 0.0224073606999229, 0.023002193742129376, 0.02379530446507154, 0.024984970549484786, 0.025579803591691264, 0.024984970549484786, 0.02538152591095587, 0.025976358953162346, 0.026571191995369114, 0.027166025037575592, 0.027959135760518047, 0.027959135760518047, 0.02875224648345963, 0.029545357206402084, 0.03033846792934425, 0.03033846792934425, 0.030933300971550726, 0.0313298563330221, 0.03212296705596397, 0.03271780009817045, 0.03291607777890643, 0.03470057690552586, 0.034502299224790464, 0.03529540994773234, 0.03668335371288127, 0.036485076032145874, 0.0380712974780302, 0.03727818675508775, 0.03787301979729481, 0.04659723774965803, 0.0406489073275918, 0.04025235196612072, 0.04005407428538532, 0.04104546268906317, 0.041442018050534254, 0.04699379311112911, 0.05155417976804641, 0.05314040121393045, 0.05333867889466584, 0.05433006729834369, 0.05452834497907909, 0.057700787870848036, 0.055718011063492626, 0.047786903834071276, 0.04461446094230262, 0.043821350219360164, 0.043821350219360164, 0.04362307253862477, 0.04421790558083154, 0.04461446094230262, 0.0452092939845091, 0.0450110163037737, 0.0452092939845091, 0.045804127026715866, 0.04600240470745155, 0.04639896006892234, 0.04719207079186451, 0.047390348472600194, 0.04798518151480696, 0.04858001455701315, 0.04937312527995531, 0.05016623600289748, 0.05135590208731072, 0.05135590208731072, 0.05135590208731072, 0.05135590208731072, 0.05155417976804641, 0.05254556817172426, 0.051752457448781805, 0.05155417976804641, 0.05214901281025318, 0.0519507351295172, 0.051752457448781805, 0.05333867889466584, 0.052347290490988574, 0.05254556817172426, 0.05294212353319505, 0.05393351193687261, 0.05393351193687261, 0.053735234256137215, 0.05393351193687261, 0.0541317896176083, 0.054726622659814775, 0.055321455702021544, 0.05551973338275694, 0.05591628874422802, 0.05710595482864156, 0.057304232509376954, 0.05849389859378991, 0.05829562091305422, 0.057700787870848036, 0.05750251019011235, 0.058097343232318535, 0.057304232509376954, 0.057700787870848036, 0.05789906555158343, 0.058097343232318535, 0.058692176274525595, 0.058692176274525595, 0.05928700931673207, 0.05948528699746776, 0.05948528699746776, 0.06087323076261669, 0.06047667540114561, 0.06047667540114561, 0.06087323076261669, 0.06087323076261669, 0.06126978612408748, 0.06126978612408748, 0.06186461916629425, 0.06245945220850073, 0.06206289684702965, 0.06186461916629425, 0.06186461916629425, 0.062261174527765334, 0.06206289684702965, 0.06206289684702965, 0.0632525629314429, 0.06285600756997181, 0.06364911829291427, 0.0630542852507072, 0.06285600756997181, 0.06245945220850073, 0.06265772988923642, 0.06285600756997181, 0.06364911829291427, 0.06384739597364966, 0.06384739597364966, 0.06384739597364966, 0.06384739597364966, 0.06464050669659183, 0.06503706205806291, 0.0652353397387986, 0.06483878437732722, 0.06543361741953399, 0.0652353397387986, 0.0652353397387986, 0.06503706205806291, 0.06563189510026968, 0.06602845046174047, 0.06682156118468263, 0.0676146719076245, 0.06880433799203804, 0.07851994434807912, 0.08149410955911209, 0.0721750585645418, 0.07138194784159993, 0.07019228175718698, 0.07019228175718698, 0.07078711479939345, 0.07019228175718698, 0.07138194784159993, 0.07197678088380641, 0.07257161392601288, 0.07237333624527749, 0.07237333624527749, 0.07356300232969074, 0.0743561130526329, 0.0743561130526329, 0.07415783537189721, 0.07415783537189721, 0.0743561130526329, 0.0745543907333683, 0.07554577913704615, 0.07415783537189721, 0.0745543907333683, 0.07554577913704615, 0.07574405681778183, 0.07594233449851723, 0.07633888985998831, 0.0767354452214591, 0.0765371675407237, 0.07633888985998831, 0.07693372290219479, 0.0765371675407237, 0.0765371675407237, 0.07614061217925233, 0.07614061217925233, 0.07614061217925233, 0.07614061217925233, 0.0765371675407237, 0.07713200058293018, 0.07693372290219479, 0.07693372290219479, 0.07733027826366587, 0.07713200058293018, 0.0765371675407237, 0.0765371675407237, 0.07614061217925233, 0.0765371675407237, 0.0765371675407237, 0.07574405681778183, 0.07554577913704615, 0.07554577913704615, 0.07475266841410427, 0.07574405681778183, 0.0745543907333683, 0.07376128001042642, 0.07356300232969074, 0.07376128001042642, 0.07336472464895534, 0.07395955769116182, 0.0743561130526329, 0.07475266841410427, 0.07495094609483967, 0.0745543907333683, 0.0743561130526329, 0.07356300232969074, 0.07257161392601288, 0.07257161392601288, 0.07376128001042642, 0.07296816928748397, 0.07276989160674857, 0.07276989160674857, 0.07276989160674857, 0.07237333624527749, 0.07257161392601288, 0.07237333624527749, 0.07197678088380641, 0.07177850320307101, 0.07158022552233533, 0.07158022552233533, 0.07177850320307101, 0.07177850320307101, 0.07237333624527749, 0.07257161392601288, 0.07276989160674857, 0.07356300232969074, 0.07356300232969074, 0.07316644696821965, 0.07376128001042642, 0.07376128001042642, 0.0743561130526329, 0.07495094609483967, 0.07554577913704615, 0.07713200058293018, 0.07752855594440126, 0.07812338898660803, 0.07871822202881451, 0.07812338898660803, 0.07832166666734372, 0.08010616579396344, 0.08684760693897126, 0.08248549796278964, 0.08149410955911209, 0.08149410955911209, 0.08169238723984748, 0.08228722028205396, 0.08724416230044234, 0.09398560344545102, 0.09339077040324396, 0.09497699184912858, 0.09596838025280614, 0.09775287937942587, 0.09834771242163234, 0.10033048922898775, 0.1017184329941364, 0.10290809907854964, 0.10469259820516966, 0.10310637675928533, 0.10310637675928533, 0.10330465444002072, 0.10409776516296318, 0.10766676341620263, 0.10786504109693802, 0.1062788196510537, 0.1104426509465002, 0.10766676341620263, 0.10905470718135127, 0.11064092862723589, 0.10905470718135127, 0.10072704459045913, 0.0991408231445748, 0.09973565618678128, 0.09953737850604588, 0.09993393386751667, 0.10013221154825236, 0.10013221154825236, 0.09973565618678128, 0.10033048922898775, 0.10033048922898775, 0.10132187763266531, 0.10132187763266531, 0.10132187763266531, 0.10132187763266531, 0.10211498835560777, 0.10211498835560777, 0.1037012098014921, 0.10270982139781425, 0.10310637675928533, 0.1037012098014921, 0.10429604284369857, 0.10409776516296318, 0.10389948748222749, 0.10469259820516966, 0.10489087588590505, 0.10528743124737643, 0.10568398660884751, 0.10588226428958261, 0.10568398660884751, 0.106080541970318, 0.10647709733178909, 0.10766676341620263, 0.1062788196510537, 0.10687365269326046, 0.10687365269326046, 0.10707193037399586, 0.10707193037399586, 0.10687365269326046, 0.10687365269326046, 0.10727020805473154, 0.10766676341620263, 0.1082615964584091, 0.10806331877767342, 0.10845987413914479, 0.10865815181988048, 0.10964954022355804, 0.11004609558502883, 0.11064092862723589, 0.11143403935017776, 0.11143403935017776, 0.11143403935017776, 0.11222715007312022, 0.11242542775385561, 0.11183059471164913, 0.11163231703091345, 0.1126237054345913, 0.11302026079606209, 0.11341681615753346, 0.11381337151900454, 0.11420992688047533, 0.11520131528415319, 0.11460648224194613, 0.1150030376034175, 0.11599442600709506, 0.11539959296488858, 0.11559787064562398, 0.11599442600709506, 0.11599442600709506, 0.11599442600709506, 0.11678753673003751, 0.11678753673003751, 0.11698581441077291, 0.11658925904930183, 0.11738236977224399, 0.11797720281445047, 0.11698581441077291, 0.11658925904930183, 0.11738236977224399, 0.11639098136856614, 0.11658925904930183, 0.1171840920915086, 0.11738236977224399, 0.11758064745297939, 0.11777892513371507, 0.1263048654053432, 0.12828764221269862, 0.11936514657959911, 0.11857203585665724, 0.1171840920915086, 0.1171840920915086, 0.11698581441077291, 0.11639098136856614, 0.11738236977224399, 0.11738236977224399, 0.11777892513371507, 0.11797720281445047, 0.11797720281445047, 0.11797720281445047, 0.11857203585665724, 0.11797720281445047, 0.11758064745297939, 0.11758064745297939, 0.1171840920915086, 0.11658925904930183, 0.11698581441077291, 0.1171840920915086, 0.11639098136856614, 0.1171840920915086, 0.11619270368783075, 0.11738236977224399, 0.11639098136856614, 0.11658925904930183, 0.11678753673003751, 0.11698581441077291, 0.11658925904930183, 0.11658925904930183, 0.11877031353739292, 0.11758064745297939, 0.11678753673003751, 0.11658925904930183, 0.11619270368783075, 0.11579614832635966, 0.11599442600709506, 0.11520131528415319, 0.11579614832635966, 0.11460648224194613, 0.11460648224194613, 0.11480475992268181, 0.11401164919973965, 0.11381337151900454, 0.11381337151900454, 0.11361509383826915, 0.11361509383826915, 0.11420992688047533, 0.11420992688047533, 0.11460648224194613, 0.11460648224194613, 0.11480475992268181, 0.11539959296488858, 0.11440820456121073, 0.11460648224194613, 0.1150030376034175, 0.11480475992268181, 0.11480475992268181, 0.1150030376034175, 0.11539959296488858, 0.11579614832635966, 0.11539959296488858, 0.11639098136856614, 0.11579614832635966, 0.11658925904930183, 0.11698581441077291, 0.11758064745297939, 0.11877031353739292, 0.11837375817592184, 0.11837375817592184, 0.11896859121812803, 0.11916686889886342, 0.11976170194107048, 0.12015825730254127, 0.12075309034474804, 0.12134792338695452, 0.12233931179063237, 0.12313242251357454, 0.12352897787504562, 0.12432208859798749, 0.12511519932092965, 0.1263048654053432, 0.1261065877246072, 0.12670142076681398, 0.12749453148975615, 0.12709797612828505, 0.12689969844754967, 0.12769280917049153, 0.12828764221269862, 0.12987386365858264, 0.12987386365858264, 0.13027041902005343, 0.13086525206226018, 0.13205491814667344, 0.1324514735081445, 0.13225319582740885, 0.13264975118887992, 0.1330463065503513, 0.13899463697241693, 0.13701186016506184, 0.1401843030568302, 0.14553780043668996, 0.1467274665211029, 0.14752057724404535, 0.14989990941287126, 0.15406374070831777, 0.15446029606978856, 0.1556499621542021, 0.1554516844734664, 0.15664135055787964, 0.15723618360008643, 0.15822757200376397, 0.15902068272670586, 0.15941723808817693, 0.1600120711303837, 0.15882240504597045, 0.15981379344964802, 0.15822757200376397, 0.15862412736523507, 0.1602103488111194, 0.1600120711303837, 0.15921896040744155, 0.16040862649185478, 0.1602103488111194, 0.15644307287714398, 0.15426201838905318, 0.1536671853468467, 0.1532706299853756, 0.15465857375052425, 0.15426201838905318, 0.15426201838905318, 0.15426201838905318, 0.15426201838905318, 0.15406374070831777, 0.15426201838905318, 0.15386546302758208, 0.153468907666111, 0.15247751926243344, 0.15247751926243344, 0.15128785317802018, 0.1508912978165491, 0.15029646477434264, 0.14970163173213585, 0.14910679868992938, 0.14930507637066479, 0.14771885492478076, 0.1445464120330121, 0.1465291888403675, 0.1495033540514002, 0.14811541028625183, 0.14712402188257429, 0.14712402188257429, 0.1469257442018383, 0.14593435579816072, 0.14712402188257429, 0.14613263347889643, 0.14494296739448287, 0.14573607811742534, 0.14573607811742534, 0.14553780043668996, 0.1467274665211029, 0.14533952275595396, 0.1447446897137475, 0.1447446897137475, 0.14494296739448287, 0.14494296739448287, 0.14533952275595396, 0.14533952275595396, 0.14553780043668996, 0.14553780043668996, 0.14573607811742534, 0.1465291888403675, 0.1467274665211029, 0.1467274665211029, 0.14593435579816072, 0.14533952275595396, 0.1465291888403675, 0.1467274665211029, 0.1469257442018383, 0.1469257442018383, 0.14633091115963182, 0.14613263347889643, 0.1467274665211029, 0.1465291888403675, 0.1467274665211029, 0.14752057724404535, 0.14771885492478076, 0.14771885492478076, 0.1485119656477229, 0.14989990941287126, 0.14989990941287126, 0.14970163173213585, 0.14989990941287126, 0.15128785317802018, 0.15168440853949128, 0.15247751926243344, 0.15267579694316913, 
